vi "ConnectIVIsampleswitch.vi"(2 "error in (no error)":errorcluster, 5 "instrument handle in":refnum<k15>) -> (0 "error out":errorcluster, 1 "instrument handle out":refnum<k15>)   [LabVIEW 2011]
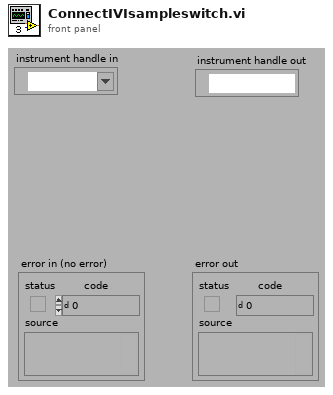
[diagram p1: front panel]
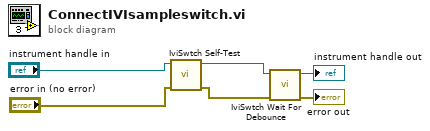
[diagram p0: block diagram]
diagram:
  n1 = call <vilib>:"IviSwtch Self-Test.vi"("error in (no error)"="error in (no error)", "instrument handle"="instrument handle in") -> ("error out"=w2:errorcluster, "instrument handle out"=w1:refnum<k15>)  [unwired: 6 in, 2 out]
  n2 = call <vilib>:"IviSwtch Wait For Debounce.vi"("error in (no error)"=w2, "instrument handle"=w1) -> ("error out"=→"error out":errorcluster, "instrument handle out"=→"instrument handle out":refnum<k15>)  [unwired: 1 in, 7 out]
